vi "Init.vi"(8 "error in":errorcluster, 11 "Combo Box in":refnum<class "Check Box.lvclass">) -> (0 "error out":errorcluster, 3 "Combo Box out":refnum<class "Check Box.lvclass">)   [LabVIEW 2024, in "SourceGrid.lvlib" / "Check Box.lvclass"]
uses:
  Check Box.lvclass
  D:/git/Sourcegrid-LabVIEW/source/Cells/Cell/Cell.lvclass
  Cell/Cell.lvclass/Cell.ctl
  D:/git/Sourcegrid-LabVIEW/dll/SourceGrid.dll
  dll/SourceGrid.dll
  Cell/Cell.lvclass
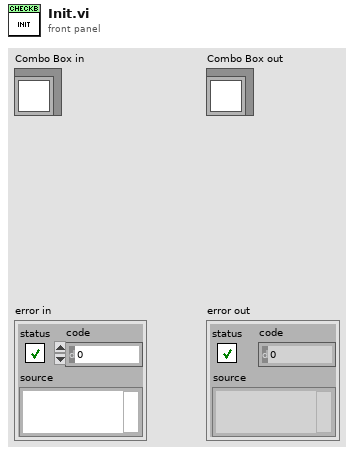
[diagram p1: front panel]
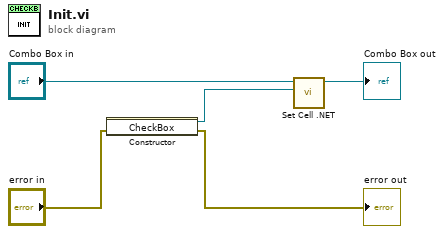
[diagram p0: block diagram]
diagram:
  n1 = constructor class="CheckBox"(error in="error in") -> (reference out=w1:refnum<k24>, error out=→"error out":errorcluster)  [unwired: 2 in, 1 out]
  n2 = call "Set Cell .NET.vi"("Cell .NET"=w1, "Cell in"="Combo Box in") -> ("Cell out"=→"Combo Box out":refnum<class "Check Box.lvclass">)  [unwired: 9 in]
